vi "Close.vi"(8 "error in (no error)":errorcluster, 11 "Log File Ref":refnum<data-value>) -> (0 "error out":errorcluster)   [LabVIEW 2014, in "Log File.lvclass"]
uses:
  Log File.lvclass
  Log File.lvclass/Log File.ctl
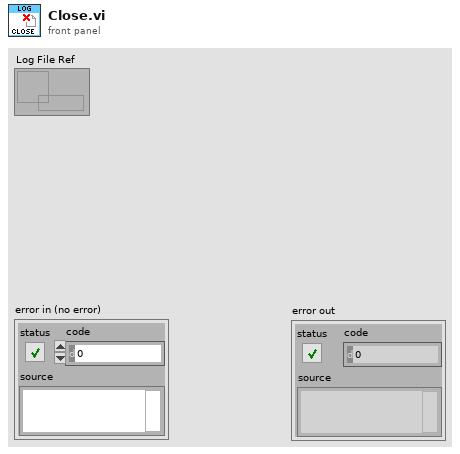
[diagram p1: front panel]
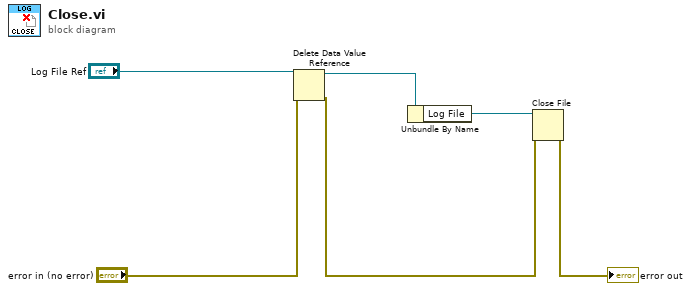
[diagram p0: block diagram]
diagram:
  n1 = Delete Data Value Reference(data value reference="Log File Ref", error in="error in (no error)") -> (data value=w4:refnum<class "Log File.lvclass">, error out=w2:errorcluster)
  n2 = Unbundle By Name(w4) -> ("Log File"=w3:refnum<file>)
  n3 = Close File(refnum=w3, error in=w2) -> (error out=→"error out":errorcluster)  [unwired: 1 out]
